vi "Initialize System.vi"(8 "error in":errorcluster, 11 "System in":refnum<class "System.lvclass">) -> (0 "error out":errorcluster, 3 "System out":refnum<class "System.lvclass">)   [LabVIEW 2014, in "System.lvclass"]
uses:
  System.lvclass
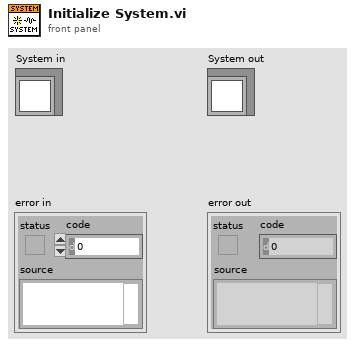
[diagram p1: front panel]
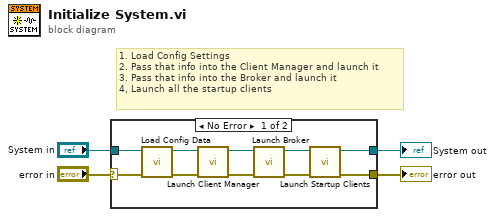
[diagram p0: block diagram]
diagram:
  # "1. Load Config Settings\n2. Pass that info into the Client Manager and launch it\n3. Pass that info into the Broker and launch it\n4, Launch all the startup clients"
  n1 = case shown="No Error" "error in" {
    selector: "error in" -> [w9 w16]
    tunnel: [w5 w16] -> w3
    tunnel: [w10 w15] -> w1
    tunnel: "System in" -> [w14 w15]
    frame No Error {
      n2 = call "Load Config Data.vi"("error in"=w9, "System in"=w14) -> ("error out"=w8:errorcluster, "System out"=w13:refnum<class "System.lvclass">)  [unwired: 8 in]
      n3 = call "Launch Client Manager.vi"("error in"=w8, "System in"=w13) -> ("error out"=w7:errorcluster, "System out"=w12:refnum<class "System.lvclass">)  [unwired: 8 in]
      n4 = call "Launch Broker.vi"("error in"=w7, "System in"=w12) -> ("error out"=w6:errorcluster, "System out"=w11:refnum<class "System.lvclass">)  [unwired: 8 in]
      n5 = call "Launch Startup Clients.vi"("error in"=w6, "System in"=w11) -> ("error out"=w5:errorcluster, "System out"=w10:refnum<class "System.lvclass">)  [unwired: 8 in]
    }
    frame Error {
    }
  }
  "error out" <- w3
  "System out" <- w1
